vi "missing_Peak3.vi"() -> ()   [LabVIEW 2016]
panel:
  out "element 2":i32
  out "element":i32
  out "Numeric 4":i32
  out "Numeric 3":i32
  out "Numeric 2":i32
  out "x+y":i32
  out "Numeric":i32
  out "array 2":i32[](array[numeric])=[0, 2, 4]
  in  "array":i32[](array[numeric])=[0, 1, 2, 4]
  out "Missing Peaks":i32[](array[numeric])
  out "Padded Peak Locations":i32[](array[numeric])=[0, 2, 4]
  in  "Average Spacing":dbl=2.0 format="%#_13g"
  in  "Width":dbl=0.1 format="%#_13g"
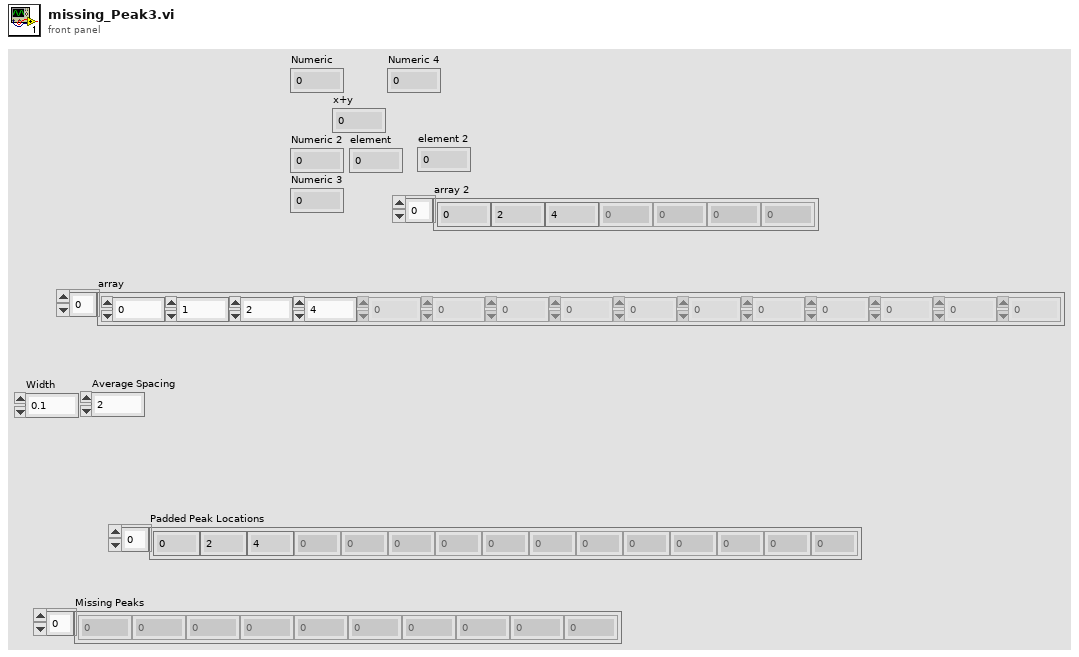
[diagram p1: front panel]
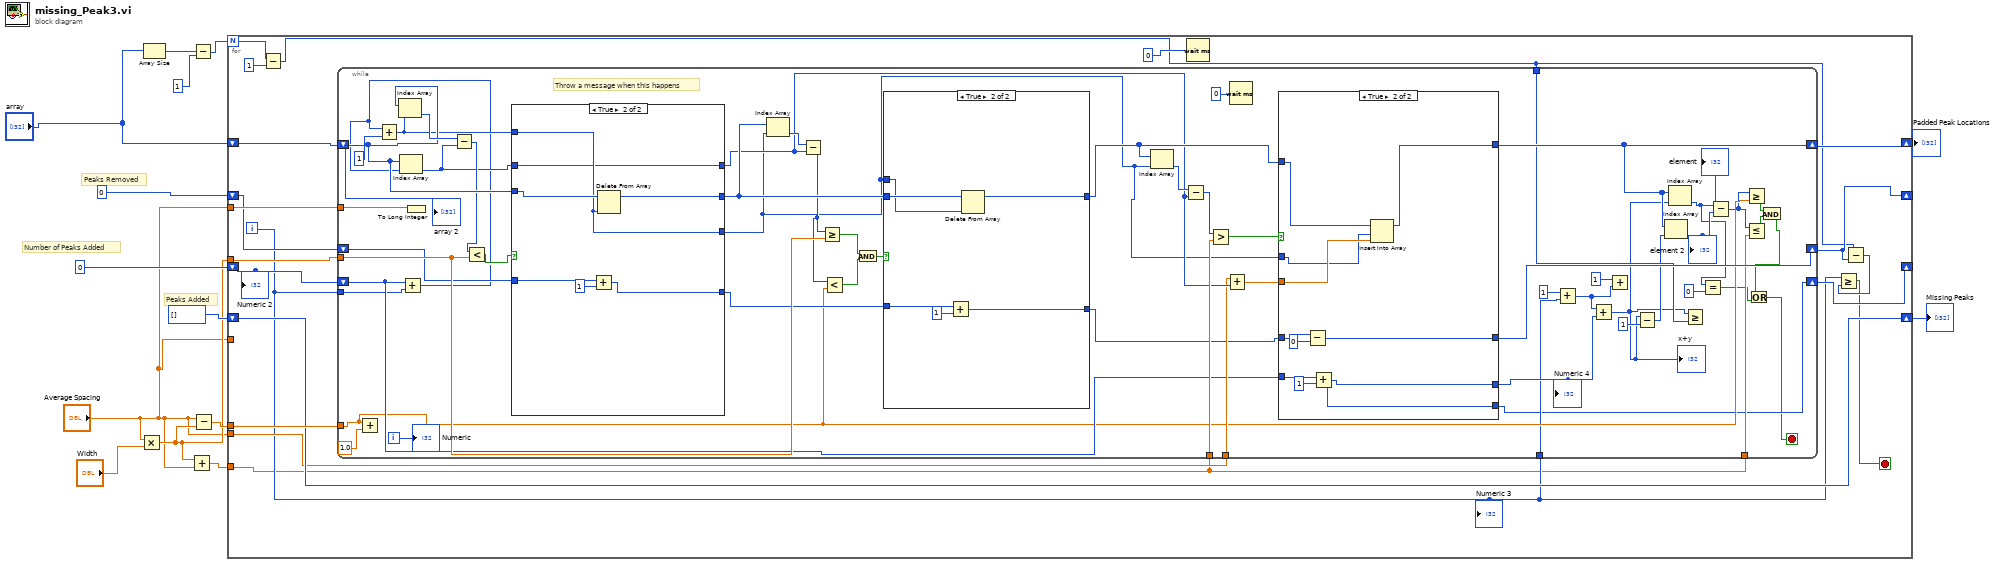
[diagram p0: block diagram]
diagram:
  # "Peaks Removed"
  # "Peaks Added"
  # "Number of Peaks Added"
  n1 = Multiply(x="Average Spacing", y="Width") -> (x*y=w3:dbl)
  n2 = Array Size(array="array") -> (size(s)=w14:i32)
  n3 = Add(x=w3, y="Average Spacing") -> (x+y=w11:dbl)
  n4 = Subtract(x=w14, y=1) -> (x-y=w12:i32)
  n5 = Subtract(x="Average Spacing", y=w3) -> (x-y=w5:dbl)
  n6 = for {
    N: w12 -> [w24]
    tunnel: w5 -> [w31]
    tunnel: w11 -> [w15]
    tunnel: "Average Spacing" -> [w33]
    shift-right: [w29] -> _
    shift-left: 0 -> [w32]
    shift-right: [w30] -> w8
    shift-left: i32[] [] ("array") -> [w30]
    tunnel: "Average Spacing" -> [_]
    tunnel: w3 -> [w28]
    shift-right: [w19] -> w4
    shift-left: "array" -> [w26]
    shift-right: [w22] -> _
    shift-left: 0 -> [w25]
    tunnel: "Average Spacing" -> [w18]
    i -> [w16]
    stop <- w20 stop-if-true
    n7 = Subtract(x=w24, y=1) -> (x-y=w17:i32)
    n8 = while {
      tunnel: w33 -> [w88]
      tunnel: w31 -> [w53]
      tunnel: w28 -> [w81]
      shift-right: [w55] -> w19
      shift-left: w26 -> [w84]
      shift-right: [w57] -> w22
      shift-left: w25 -> [w72]
      tunnel: w15 -> [w68]
      tunnel: w18 -> [w63]
      shift-right: [w48] -> w29
      shift-left: w32 -> [w60]
      tunnel: w16 -> [w59]
      tunnel: w17 -> [w39]
      tunnel: w16 -> [w51]
      tunnel: w15 -> [w54]
      i -> [w49]
      stop <- w41 stop-if-true
      # "Throw a message when this happens"
      n9 = Add(x=w53, y=1.0) -> ()  [unwired: 1 out]
      n10 = Add(x=w60, y=w59) -> (x+y=w58:i32)
      n11 = Add(x=w58, y=1) -> (x+y=w83:i32)
      n12 = Index Array(array=w84, index=w83) -> (element=w85:i32)
      n13 = Index Array(array=w84, index=w58) -> (element=w73:i32)
      n14 = To Long Integer(number=w88) -> ()  [unwired: 1 out]
      n15 = Subtract(x=w85, y=w73) -> (x-y=w82:i32)
      n16 = Less?(x=w82, y=w81) -> (x < y?=w86:bool)
      n17 = case shown="True" w86 {
        tunnel: w84 -> [w114 w121]
        tunnel: w83 -> [w113 w119]
        tunnel: [w114 w120] -> w77
        tunnel: [w113 w119] -> w62
        tunnel: w73 -> [w112 w118]
        tunnel: [w112 w118] -> w64
        tunnel: w72 -> [w111 w117]
        tunnel: [w111 w116] -> w71
        frame False {
        }
        frame True {
          n18 = Add(x=w117, y=1) -> (x+y=w116:i32)
          n19 = Delete From Array(array=w121, index=w119) -> (array with subset deleted=w120:i32[])  [unwired: 1 in, 1 out]
        }
      }
      n20 = Index Array(array=w77, index=w62) -> (element=w75:i32)
      n21 = Subtract(x=w75, y=w64) -> (x-y=w76:i32)
      n22 = Greater Or Equal?(x=w76, y=w81) -> (x >= y?=w80:bool)
      n23 = Less?(x=w76, y=w53) -> (x < y?=w79:bool)
      n24 = And(x=w80, y=w79) -> (x .and. y?=w78:bool)
      n25 = case shown="True" w78 {
        tunnel: w77 -> [w104 w110]
        tunnel: [w104 w109] -> w66
        tunnel: w62 -> [_ w108]
        tunnel: w71 -> [w103 w107]
        tunnel: [w103 w105] -> w61
        frame False {
        }
        frame True {
          n26 = Add(x=w107, y=1) -> (x+y=w105:i32)
          n27 = Delete From Array(array=w110, index=w108) -> (array with subset deleted=w109:i32[])  [unwired: 1 in, 1 out]
        }
      }
      n28 = Index Array(array=w66, index=w62) -> (element=w70:i32)
      n29 = Subtract(x=w70, y=w64) -> (x-y=w69:i32)
      n30 = Greater?(x=w69, y=w68) -> (0:w67:bool)
      n31 = Add(x=w63, y=w64) -> (x+y=w65:dbl)
      n32 = Wait (ms)(milliseconds to wait=u32 0) -> ()  [unwired: 1 out]
      n33 = case shown="True" w67 {
        tunnel: w66 -> [w92 w102]
        tunnel: [w92 w101] -> w55
        tunnel: w65 -> [_ w100]
        tunnel: w62 -> [_ w99]
        tunnel: w61 -> [w91 w98]
        tunnel: [w91 w96] -> w57
        tunnel: w60 -> [w90 w94]
        tunnel: [w90 w93] -> w52
        tunnel: [w90 w93] -> w48
        frame False {
        }
        frame True {
          n34 = Subtract(x=w98, y=0) -> (x-y=w96:i32)
          n35 = Add(x=w94, y=1) -> (x+y=w93:i32)
          n36 = Insert Into Array(array=w102, index=w99, new element=w100) -> (w101:i32[])
        }
      }
      "Numeric 4" <- w52
      n37 = Add(x=1, y=w51) -> (x+y=w36:i32)
      n38 = Add(x=w36, y=w52) -> (x+y=w35:i32)
      "x+y" <- w35
      n39 = Add(x=1, y=w36) -> ()  [unwired: 1 out]
      n40 = Subtract(x=w35, y=1) -> (x-y=w37:i32)
      n41 = Index Array(array=w55, index=w37) -> (element=w47:i32)
      "element 2" <- w47
      n42 = Index Array(array=w55, index=w35) -> (element=w43:i32)
      "element" <- w43
      n43 = Greater Or Equal?(x=w35, y=w39) -> ()  [unwired: 1 out]
      n44 = Equal?(x=w43, y=0) -> (x = y?=w34:bool)
      n45 = Subtract(x=w43, y=w47) -> (x-y=w46:i32)
      n46 = Greater Or Equal?(x=w46, y=w53) -> (x >= y?=w45:bool)
      n47 = Less Or Equal?(x=w46, y=w54) -> (x <= y?=w44:bool)
      n48 = And(x=w45, y=w44) -> (x .and. y?=w42:bool)
      n49 = Or(x=w42, y=w34) -> (x .or. y?=w41:bool)
      "array 2" <- w84
      "Numeric" <- w49
    }
    n50 = Wait (ms)(milliseconds to wait=u32 0) -> ()  [unwired: 1 out]
    n51 = Subtract(x=w17, y=w22) -> (x-y=w21:i32)
    n52 = Greater Or Equal?(x=w16, y=w21) -> (x >= y?=w20:bool)
    "Numeric 2" <- w32
    "Numeric 3" <- w16
  }
  "Padded Peak Locations" <- w4
  "Missing Peaks" <- w8
